vi "tempconfigbinfileIp.vi"(1 "Temp Config in":T2, 2 "command":string) -> (0 "Temp Config out":T1)   [LabVIEW 2015]
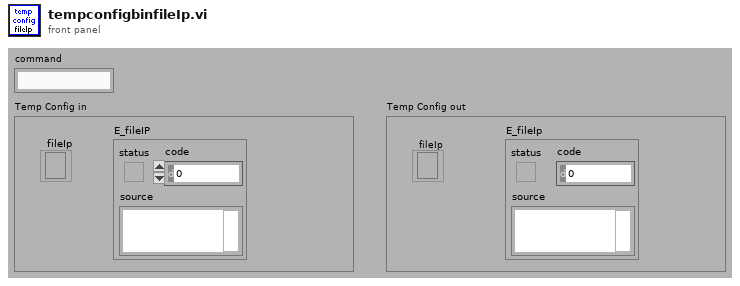
[diagram p1: front panel]
types:
  T1 = cluster{"fileIp":refnum<file>, "E_fileIp":errorcluster}
  T2 = cluster{"fileIp":refnum<file>, "E_fileIP":errorcluster}
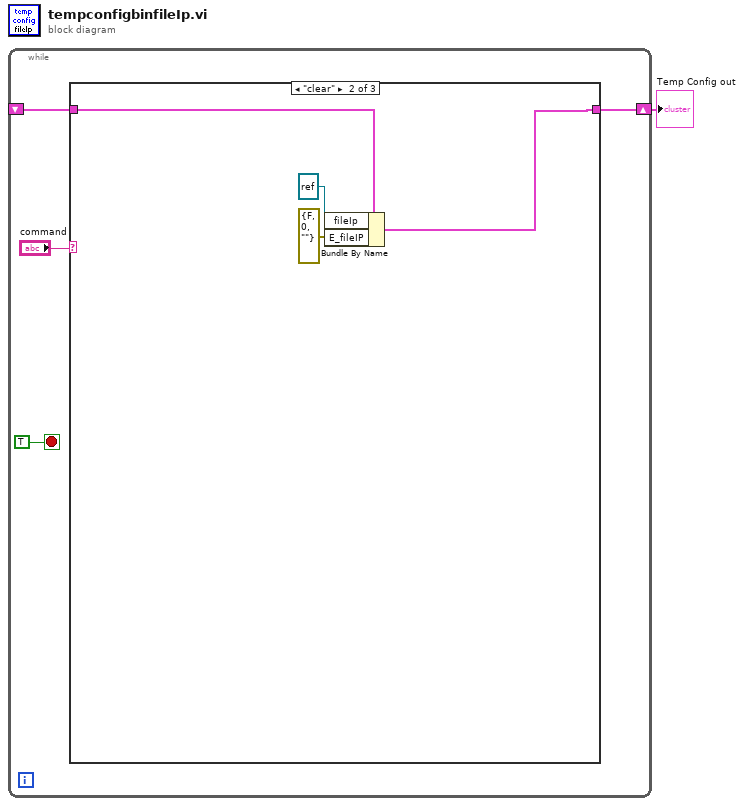
[diagram p0: block diagram]
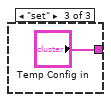
[diagram p3: hidden frame]
diagram:
  n1 = while {
    shift-right: [w3] -> w1
    shift-left: _ -> [w2]
    stop <- TRUE stop-if-true
    n2 = case shown="\"clear\"" "command" {
      tunnel: [w6 w9 "Temp Config in"] -> w3
      tunnel: w2 -> [w6 w10 _]
      frame "get", Default {
      }
      frame "clear" {
        n3 = Bundle By Name(cluster=w10, "fileIp"=refnum<file> refnum ("refnum tif 1"), "E_fileIP"=errorcluster {"status"=FALSE, "code"=0, "source"=""} ("E_tif0")) -> (w9:T2)
      }
      frame "set" {
      }
    }
  }
  "Temp Config out" <- w1
